vi "Waveform Graph.vi"() -> ()   [LabVIEW 2023]
panel:
  out "Waveform Graph":dbl[][](graph)
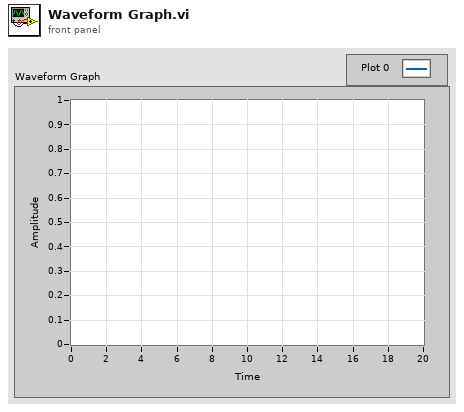
[diagram p1: front panel]
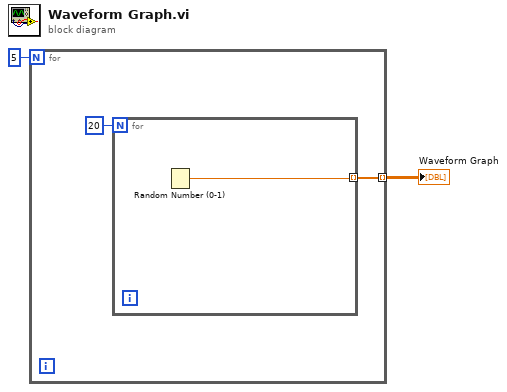
[diagram p0: block diagram]
diagram:
  n1 = for {
    N: 5 -> [_]
    tunnel: [w4] -> w2 mode=indexing
    n2 = for {
      N: 20 -> [_]
      tunnel: [w5] -> w4 mode=indexing
      n3 = Random Number (0-1)() -> (number: 0 to 1=w5:dbl)
    }
  }
  "Waveform Graph" <- w2
